vi "Drawing Debug.vi"() -> ()   [LabVIEW 2021]
uses:
  <vilib>/BLE/type_def/address_type.ctl
  <vilib>/BLE/type_def/connection_status_bundle.ctl
  <vilib>/Utility/inputDevices.llb/closeJoystick.vi
  <vilib>/Utility/inputDevices.llb/mouseAcquire.vi
  <vilib>/BLE/ble_functions/ble_write_by_service_characteristic_uint8array.vi
panel:
  out "Connected":bool
  out "Device Name":string
  out "Handle table":string[][](array[string])
  out "Connection Status":T1={"MAC Address"="", "cnx handle"=0, "cnx flags"=0, "Address Type"=125, "Connection Interval (ms)"=125, "Timeout(ms)"=125, "Latency"=0, "bonding handle"=0} {"Address Type" items=["Public", "Random"]}
  out "Scanning":bool
  in  "Continue":bool
  in  "MAC Address":string="00:A0:50:9A:94:D6"
  in  "Address Type":T2=1 items=["Public", "Random"]
  in  "COM Bluegiga in":refnum<visa-resource-name>="COM5"
  out "Devices":string[][](array[string])
  out "BLED112 Dongle Info":string
  in  "Scale: mm per pixel":u32=1 min=1 max=10
  in  "Clear Drawing":bool
  out "Robot Drawn So Far":cluster{i32[], i32[]}[](graph)
  in  "Cancel Drawing Queue":bool
  out "Obstacle Detected":bool
  out "Robot Vertical":dbl
  out "Robot Horizontal":dbl
  out "Chalk Force Readout":dbl
  out "Current Mouse Coordinates":T3
  out "Drawing":cluster{i32[], i32[]}[](graph)
  out "Mouse Status":cluster{"Clicked?":bool}
  in  "Emergency Stop":bool
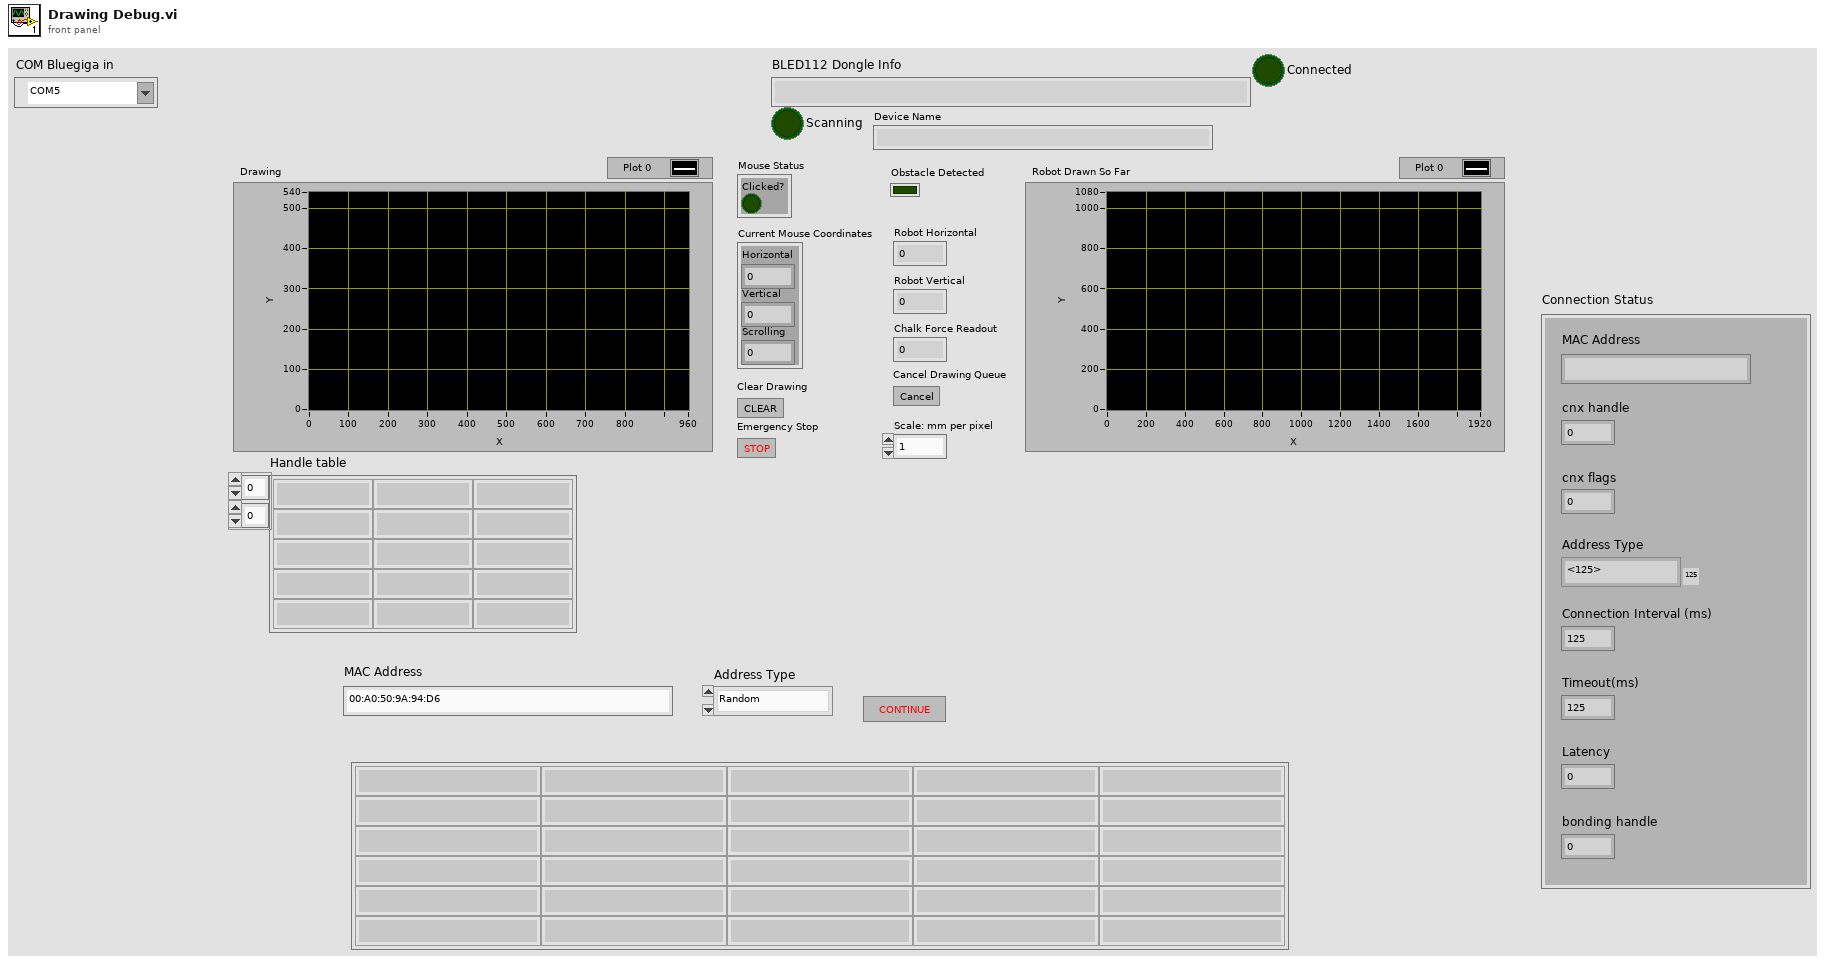
[diagram p1: front panel]
types:
  T1 = typedef "connection_status_bundle.ctl" = cluster{"MAC Address":string, "cnx handle":u8, "cnx flags":u8, "Address Type":T2, "Connection Interval (ms)":u16, "Timeout(ms)":u16, "Latency":u16, "bonding handle":u8}
  T2 = typedef "address_type.ctl" = u8
  T3 = cluster{"Horizontal":i32, "Vertical":i32, "Scrolling":i32}
  T4 = cluster{"Horizontal Array":i32[], "Vertical Array":i32[]}
  T5 = cluster{"Horizontal Array":i32[], "Vertical Array":i32[]}[]
  T6 = cluster{"button 1":bool, "button 2":bool, "button 3":bool, "button 4":bool}
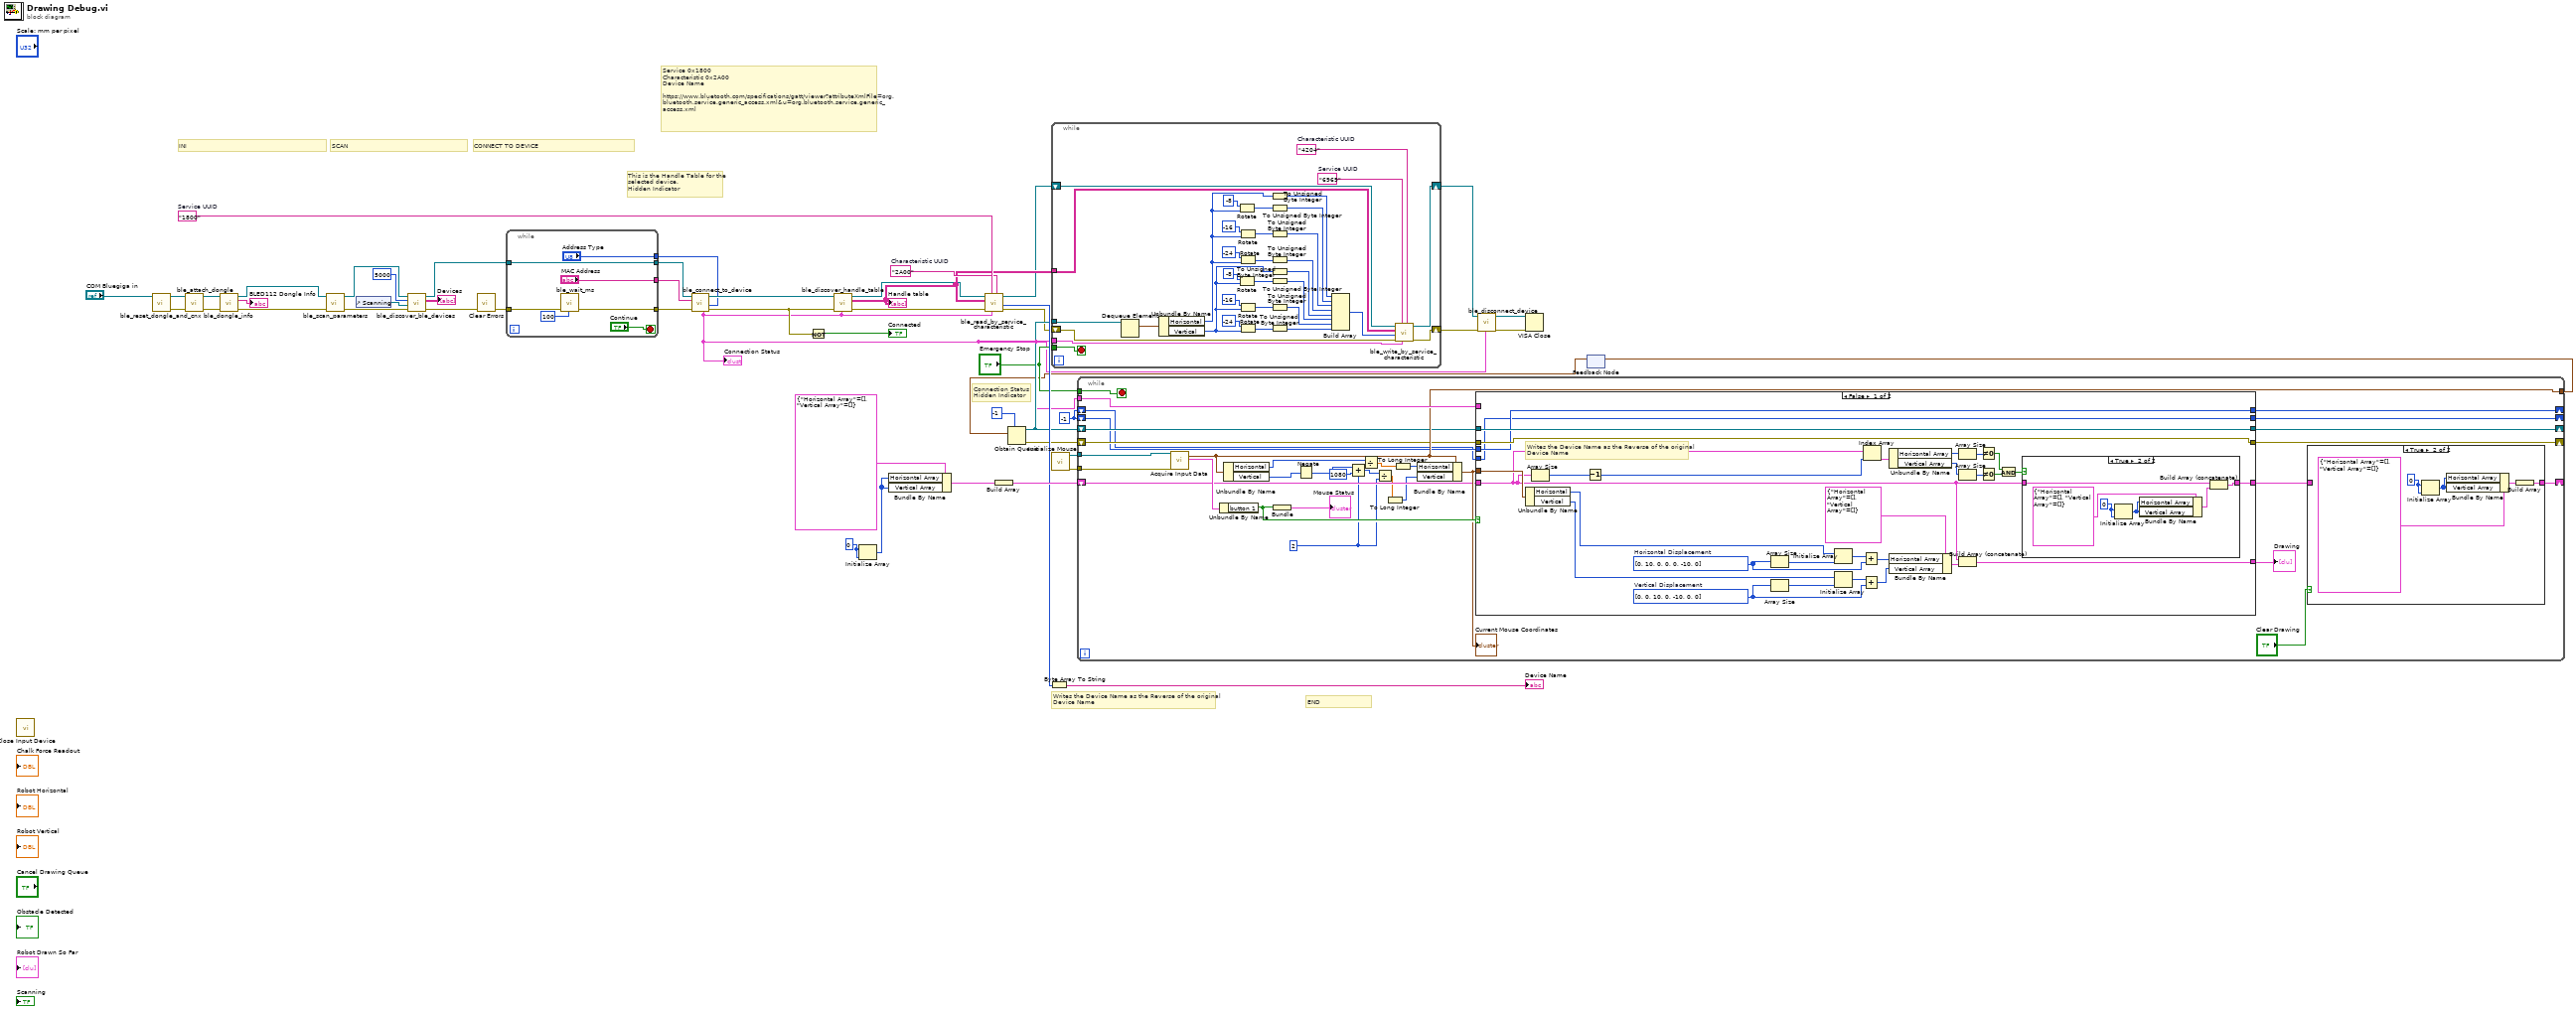
[diagram p0: block diagram]
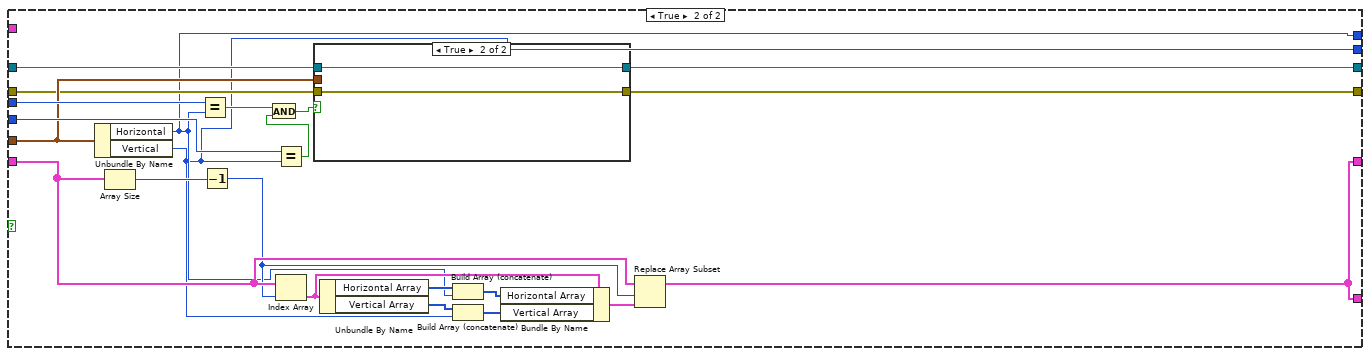
[diagram p4: hidden frame]
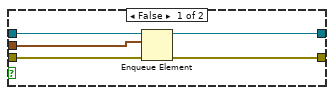
[diagram p5: hidden frame]
diagram:
  w1 = -1
  w14 = "2A00"  # Characteristic UUID
  w16 = "1800"  # Service UUID
  w47 = 0
  # "Writes the Device Name as the Reverse of the original\nDevice Name"
  # "Connection Status\nHidden Indicator"
  # "Service 0x1800\nCharacteristic 0x2A00\nDevice Name\n\nhttps://www.bluetooth.com/specifications/gatt/viewer?attributeXmlFile=org.bluetooth.service.generic_access.xml&u=org.bluetooth.service.generic_access.xml"
  # "This is the Handle Table for the\nselected device. \nHidden Indicator"
  # "CONNECT TO DEVICE"
  # "SCAN"
  # "END"
  # "INI"
  n1 = call-poly <vilib>:"Close Input Device.vi"() -> ()  [unwired: 10 in, 1 out]
  n2 = call <vilib>:"ble_reset_dongle_and_cnx.vi"("COM Bluegiga in"="COM Bluegiga in") -> ("error out"=w28:errorcluster, "COM Bluegiga out"=w26:refnum<visa-resource-name>)  [unwired: 9 in]
  n3 = call <vilib>:"ble_attach_dongle.vi"("error in (no error)"=w28, "COM Bluegiga in"=w26) -> ("error out"=w30:errorcluster, "COM Bluegiga out"=w29:refnum<visa-resource-name>)  [unwired: 8 in]
  n4 = call <vilib>:"ble_dongle_info.vi"("error in (no error)"=w30, "COM Bluegiga in"=w29) -> ("error out"=w36:errorcluster, "info"=→"BLED112 Dongle Info":string, "COM Bluegiga out"=w37:refnum<visa-resource-name>)  [unwired: 7 in]
  n5 = call <vilib>:"ble_scan_parameters.vi"("error in (no error)"=w36, "COM Bluegiga in"=w37) -> ("error out"=w34:errorcluster, "COM Bluegiga out"=w35:refnum<visa-resource-name>)  [unwired: 7 in, 1 out]
  n6 = control-ref of="Scanning"() -> (w40:refnum<vi>)
  n7 = call <vilib>:"ble_discover_ble_devices.vi"("error in (no error)"=w34, "LED ref"=w40, "Scan Duration (10000ms)"=u32 5000, "COM Bluegiga in"=w35) -> ("error out"=w24:errorcluster, "Devices"=→"Devices":string[][], "COM Bluegiga out"=w41:refnum<visa-resource-name>)  [unwired: 5 in]
  n8 = call <vilib>:"Clear Errors.vi"("error in (no error)"=w24) -> ("error out"=w23:errorcluster)  [unwired: 5 in, 1 out]
  n9 = while {
    tunnel: w23 -> [w57]
    tunnel: [w56] -> w39
    tunnel: w41 -> [w56]
    tunnel: [w55] -> w38
    tunnel: ["MAC Address"] -> w31
    tunnel: ["Address Type"] -> w22
    stop <- "Continue" stop-if-true
    n10 = call <vilib>:"ble_wait_ms.vi"("milliseconds to wait (100)"=u32 100, "error in (no error)"=w57) -> ("error out"=w55:errorcluster)  [unwired: 9 in]
  }
  n11 = call <vilib>:"ble_connect_to_device.vi"("Address Type"=w22, "error in (no error)"=w38, "MAC Address"=w31, "COM Bluegiga in"=w39) -> ("error out"=w17:errorcluster, "COM Bluegiga out"=w25:refnum<visa-resource-name>, "Connection Status"=w9:T1)  [unwired: 5 in]
  "Connection Status" <- w9
  n12 = Not(x=w17) -> (.not. x?=→"Connected":bool)
  n13 = call <vilib>:"ble_discover_handle_table.vi"("Connection Status"=w9, "error in (no error)"=w17, "COM Bluegiga in"=w25) -> ("error out"=w21:errorcluster, "Handle table"=w8:string[][], "COM Bluegiga out"=w20:refnum<visa-resource-name>)  [unwired: 6 in]
  "Handle table" <- w8
  n14 = Initialize Array(w47, w47) -> (w45:i32[])
  n15 = Bundle By Name(cluster=T4 {"Horizontal Array"=[], "Vertical Array"=[]}, "Horizontal Array"=w45, "Vertical Array"=w45) -> (w48:T4)
  n16 = call <vilib>:"ble_read_by_service_characteristic.vi"("Characteristic UUID"=w14, "Connection Status"=w9, "Service UUID"=w16, "error in (no error)"=w21, "Handle table"=w8, "COM Bluegiga in"=w20) -> ("error out"=w6:errorcluster, "attribute value"=w15:u8[], "COM Bluegiga out"=w7:refnum<visa-resource-name>)  [unwired: 2 in, 1 out]
  n17 = Build Array(w48) -> (w46:T5)
  n18 = Byte Array To String(unsigned byte array=w15) -> (string=→"Device Name":string)
  n19 = call <vilib>:"Initialize Mouse.vi"() -> ("error out"=w50:errorcluster, "device ID"=w51:refnum<k1>)  [unwired: 10 in]
  n20 = feedback #1() -> (w2:T3)  [unwired: 1 in]
  n21 = Obtain Queue(max queue size (-1, unlimited)=-1, element data type=w2) -> (queue out=w11:refnum<queue>, error out=w12:errorcluster)  [unwired: 3 in, 1 out]
  n22 = while {
    tunnel: w11 -> [w69]
    tunnel: "Emergency Stop" -> [w65]
    tunnel: w9 -> [w64]
    tunnel: w8 -> [w63]
    shift-right: [w61] -> w4
    shift-left: w7 -> [w62]
    shift-right: [w59] -> w5
    shift-left: w6 -> [w60]
    stop <- w65 stop-if-true
    w91 = "6969"  # Service UUID
    w92 = "4204"  # Characteristic UUID
    n23 = Dequeue Element(queue=w69) -> (element=w68:T3)  [unwired: 2 in, 3 out]
    n24 = Unbundle By Name(w68) -> ("Horizontal"=w67:i32, "Vertical"=w66:i32)
    n25 = Rotate(1:w67, 2:-8) -> (0:w81:i32)
    n26 = Rotate(1:w66, 2:-8) -> (0:w84:i32)
    n27 = Rotate(1:w67, 2:-16) -> (0:w82:i32)
    n28 = Rotate(1:w67, 2:-24) -> (0:w83:i32)
    n29 = Rotate(1:w66, 2:-16) -> (0:w85:i32)
    n30 = Rotate(1:w66, 2:-24) -> (0:w86:i32)
    n31 = To Unsigned Byte Integer(number=w67) -> (unsigned 8bit integer=w77:u8)
    n32 = To Unsigned Byte Integer(number=w81) -> (unsigned 8bit integer=w80:u8)
    n33 = To Unsigned Byte Integer(number=w82) -> (unsigned 8bit integer=w79:u8)
    n34 = To Unsigned Byte Integer(number=w83) -> (unsigned 8bit integer=w78:u8)
    n35 = To Unsigned Byte Integer(number=w66) -> (unsigned 8bit integer=w87:u8)
    n36 = To Unsigned Byte Integer(number=w84) -> (unsigned 8bit integer=w88:u8)
    n37 = To Unsigned Byte Integer(number=w85) -> (unsigned 8bit integer=w89:u8)
    n38 = To Unsigned Byte Integer(number=w86) -> (unsigned 8bit integer=w90:u8)
    n39 = Build Array(w77, w80, w79, w78, w87, w88, w89, w90) -> (w70:u8[])
    n40 = call-poly <vilib>:"ble_write_by_service_characteristic.vi"("Characteristic UUID"=w92, "Connection Status"=w64, "Service UUID"=w91, "error in (no error)"=w60, "data"=w70, "Handle table"=w63, "COM Bluegiga in"=w62) -> ("error out"=w59:errorcluster, "COM Bluegiga out"=w61:refnum<visa-resource-name>)  [unwired: 3 in]
  }
  n41 = while {
    tunnel: w51 -> [w124]
    tunnel: w50 -> [w123]
    shift-right: [w113] -> _
    shift-left: w46 -> [w117]
    tunnel: w9 -> [w112]
    tunnel: [w109] -> w3
    shift-right: [w105] -> _
    shift-left: w11 -> [w108]
    shift-right: [w106] -> _
    shift-left: w12 -> [w107]
    tunnel: "Emergency Stop" -> [w104]
    shift-right: [w101] -> _
    shift-left: w1 -> [w103]
    shift-right: [w100] -> _
    shift-left: w1 -> [w102]
    stop <- w104 stop-if-true
    w95 = 2
    n42 = call-poly <vilib>:"Acquire Input Data.vi"("device ID"=w124, "error in (no error)"=w123) -> ("axis info"=w109:T3, "button info"=w122:T6)  [unwired: 14 in, 2 out]
    n43 = Unbundle By Name(w122) -> ("button 1"=w119:bool)
    n44 = Unbundle By Name(w109) -> ("Horizontal"=w96:i32, "Vertical"=w121:i32)
    n45 = Bundle("button 1"=w119) -> (→"Mouse Status":cluster{"button 1":bool})  [unwired: 1 in]
    n46 = Negate(x=w121) -> (-x=w111:i32)
    n47 = Add(x=w111, y=1080) -> (x+y=w97:i32)
    n48 = Divide(x=w96, y=w95) -> (x/y=w93:dbl)
    n49 = Divide(x=w97, y=w95) -> (x/y=w99:dbl)
    n50 = To Long Integer(number=w99) -> (32bit integer=w98:i32)
    n51 = To Long Integer(number=w93) -> (32bit integer=w94:i32)
    n52 = Bundle By Name(cluster=w109, "Horizontal"=w94, "Vertical"=w98) -> (w118:T3)
    "Current Mouse Coordinates" <- w118
    n53 = case shown="False" w119 {
      tunnel: w117 -> [w147 w183]
      tunnel: w118 -> [w149 w175]
      tunnel: [w150 w180] -> w114
      tunnel: [w145 w180] -> w116
      tunnel: w112 -> [_ _]
      tunnel: w108 -> [w134 w171]
      tunnel: w107 -> [w133 w174]
      tunnel: [w133 w172] -> w106
      tunnel: [w134 w173] -> w105
      tunnel: w103 -> [w132 w178]
      tunnel: w102 -> [w131 w177]
      tunnel: [w132 w169] -> w101
      tunnel: [w131 w168] -> w100
      frame False {
        w139 = i32[] [0, 0, 10, 0, -10, 0, 0]  # Vertical Displacement
        w141 = i32[] [0, 10, 0, 0, 0, -10, 0]  # Horizontal Displacement
        # "Writes the Device Name as the Reverse of the original\nDevice Name"
        n54 = Unbundle By Name(w149) -> ("Horizontal"=w136:i32, "Vertical"=w135:i32)
        n55 = Array Size(array=w147) -> (size(s)=w158:i32)
        n56 = Decrement(x=w158) -> (x-1=w160:i32)
        n57 = Array Size(array=w141) -> (size(s)=w144:i32)
        n58 = Array Size(array=w139) -> (size(s)=w143:i32)
        n59 = Initialize Array(w136, w144) -> (w142:i32[])
        n60 = Initialize Array(w135, w143) -> (w140:i32[])
        n61 = Add(x=w142, y=w141) -> (x+y=w137:i32[])
        n62 = Add(x=w140, y=w139) -> (x+y=w138:i32[])
        n63 = Index Array(array=w147, index=w160) -> (element=w159:T4)
        n64 = Unbundle By Name(w159) -> ("Horizontal Array"=w157:i32[], "Vertical Array"=w156:i32[])
        n65 = Bundle By Name(cluster=T4 {"Horizontal Array"=[], "Vertical Array"=[]}, "Horizontal Array"=w137, "Vertical Array"=w138) -> (w146:T4)
        n66 = Array Size(array=w157) -> (size(s)=w155:i32)
        n67 = Array Size(array=w156) -> (size(s)=w154:i32)
        n68 = Build Array (concatenate)(w147, w146) -> (w145:T5)
        n69 = Not Equal To 0?(x=w155) -> (x != 0?=w153:bool)
        n70 = Not Equal To 0?(x=w154) -> (x != 0?=w152:bool)
        n71 = And(x=w153, y=w152) -> (x .and. y?=w151:bool)
        n72 = case shown="True" w151 {
          tunnel: w147 -> [w161 w165]
          tunnel: [w161 w162] -> w150
          frame False {
          }
          frame True {
            w166 = 0
            n73 = Initialize Array(w166, w166) -> (w167:i32[])
            n74 = Bundle By Name(cluster=T4 {"Horizontal Array"=[], "Vertical Array"=[]}, "Horizontal Array"=w167, "Vertical Array"=w167) -> (w163:T4)
            n75 = Build Array (concatenate)(w165, w163) -> (w162:T5)
          }
        }
      }
      frame True {
        n76 = Unbundle By Name(w175) -> ("Horizontal"=w169:i32, "Vertical"=w168:i32)
        n77 = Array Size(array=w183) -> (size(s)=w189:i32)
        n78 = Equal?(x=w178, y=w169) -> (x = y?=w179:bool)
        n79 = Decrement(x=w189) -> (x-1=w182:i32)
        n80 = Equal?(x=w177, y=w168) -> (x = y?=w176:bool)
        n81 = And(x=w179, y=w176) -> (x .and. y?=w170:bool)
        n82 = Index Array(array=w183, index=w182) -> (element=w186:T4)
        n83 = case shown="True" w170 {
          tunnel: w175 -> [w194 _]
          tunnel: w174 -> [w193 w195]
          tunnel: [w192 w196] -> w173
          tunnel: [w191 w195] -> w172
          tunnel: w171 -> [w190 w196]
          frame False {
            n84 = Enqueue Element(queue=w190, element=w194, error in (no error)=w193) -> (queue out=w192:refnum<queue>, error out=w191:errorcluster)  [unwired: 1 in, 1 out]
          }
          frame True {
          }
        }
        n85 = Unbundle By Name(w186) -> ("Horizontal Array"=w188:i32[], "Vertical Array"=w187:i32[])
        n86 = Build Array (concatenate)(w188, w169) -> (w185:i32[])
        n87 = Build Array (concatenate)(w187, w168) -> (w184:i32[])
        n88 = Bundle By Name(cluster=w186, "Horizontal Array"=w185, "Vertical Array"=w184) -> (w181:T4)
        n89 = Replace Array Subset(array=w183, new element=w181, index=w182) -> (w180:T5)
      }
    }
    "Drawing" <- w116
    n90 = case shown="True" "Clear Drawing" {
      tunnel: w114 -> [w125 _]
      tunnel: [w125 w126] -> w113
      frame False {
      }
      frame True {
        w128 = 0
        n91 = Initialize Array(w128, w128) -> (w130:i32[])
        n92 = Bundle By Name(cluster=T4 {"Horizontal Array"=[], "Vertical Array"=[]}, "Horizontal Array"=w130, "Vertical Array"=w130) -> (w129:T4)
        n93 = Build Array(w129) -> (w126:T5)
      }
    }
  }
  n94 = call <vilib>:"ble_disconnect_device.vi"("Connection Status"=w9, "error in (no error)"=w5, "COM Bluegiga in"=w4) -> ("error out"=w32:errorcluster, "COM Bluegiga out"=w33:refnum<visa-resource-name>)  [unwired: 7 in]
  n95 = VISA Close(VISA resource name=w33, error in (no error)=w32) -> ()  [unwired: 1 out]
  n96 = feedback-in #1(w3) -> ()
